vi "SFTF_attractor.vi"(10 "Target_Flash_Order":i64[](array[numeric]), 11 "Brain_EEG":dbl[][](array[numeric])) -> (2 "Non STFT":dbl[](array[numeric]), 3 "STFT Spectrogram {X}":dbl[][](array[numeric]))   [LabVIEW 2014]
uses:
  <vilib>/Analysis/3filter.llb/Filter Passband Type.ctl
  <vilib>/Analysis/4window.llb/windowTd.ctl
  <vilib>/Analysis/3filter.llb/Butterworth Filter (DBL).vi
  <vilib>/Analysis/NI_AALBase.lvlib
  <vilib>/gmath/NI_Gmath.lvlib
  <vilib>/Analysis/NI_AALPro.lvlib
panel:
  out "size(s)":i32
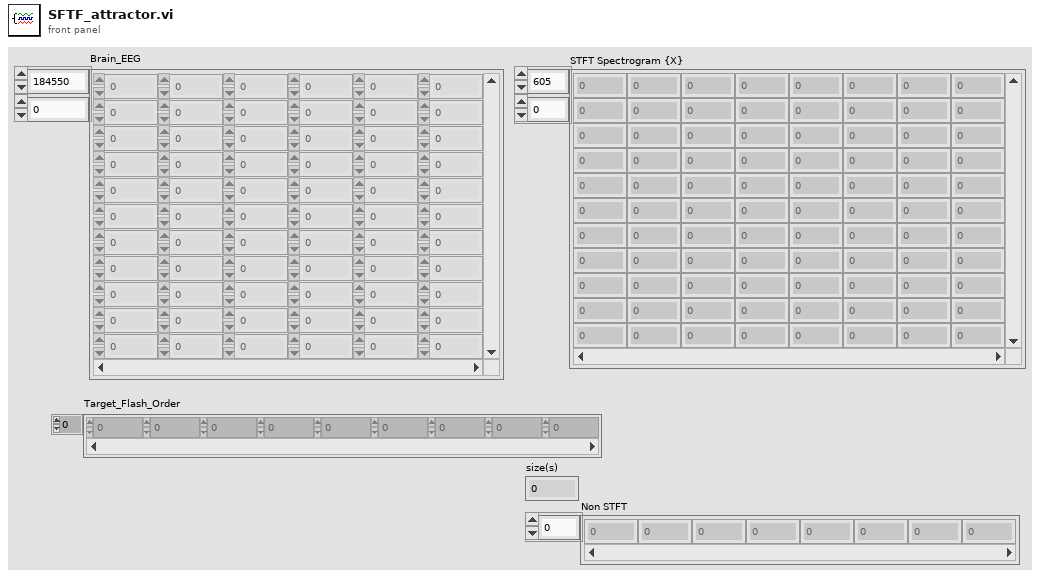
[diagram p1: front panel]
types:
  T1 = typedef "NI_AALPro.lvlib/windowTd.ctl" = u32
  T2 = typedef "NI_AALBase.lvlib/Filter Passband Type.ctl" = enum32{"Lowpass", "Highpass", "Bandpass", "Bandstop"}
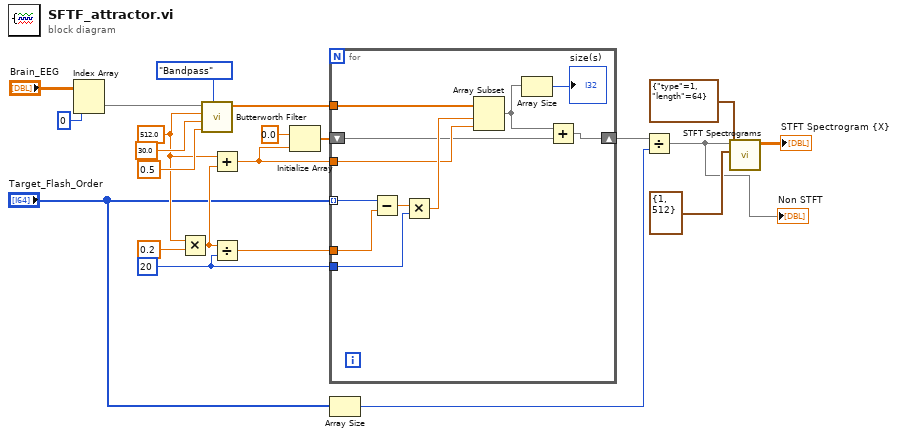
[diagram p0: block diagram]
diagram:
  w14 = 20 ("high cutoff freq: fh")
  w13 = 512.0 ("high cutoff freq: fh")
  n1 = Index Array(array="Brain_EEG", index (col)=0 ("disabled index (col)")) -> (element=w17:dbl[])  [unwired: 1 in]
  n2 = Multiply(x=w13, y=0.2) -> (x*y=w12:dbl)
  n3 = call-poly <vilib>:"Butterworth Filter.vi"("filter type"=Filter_Passband_Type."Bandpass", "low cutoff freq: fl"=0.5, "high cutoff freq: fh"=30.0, "sampling freq: fs"=w13, "X"=w17) -> ("Filtered X"=w2:dbl[])  [unwired: 3 in, 1 out]
  n4 = Add(x=w13, y=w12) -> (x+y=w10:dbl)
  n5 = Divide(x=w12, y=w14) -> (x/y=w15:dbl)
  n6 = Initialize Array(0.0 ("element"), w10) -> (w9:dbl[])
  n7 = for {
    tunnel: w2 -> [w31]
    tunnel: "Target_Flash_Order" -> [w30] mode=indexing
    tunnel: w15 -> [w29]
    tunnel: w14 -> [w28]
    tunnel: w10 -> [w27]
    shift-right: [w25] -> w8
    shift-left: w9 -> [w26]
    n8 = Subtract(x=w30, y=w29) -> (x-y=w33:dbl)
    n9 = Multiply(x=w33, y=w28) -> (x*y=w32:dbl)
    n10 = Array Subset(array=w31, index=w32, length=w27) -> (w23:dbl[])
    n11 = Array Size(array=w23) -> (size(s)=→"size(s)":i32)
    n12 = Add(x=w23, y=w26) -> (x+y=w25:dbl[])
  }
  n13 = Array Size(array="Target_Flash_Order") -> (size(s)=w7:i32)
  n14 = Divide(x=w8, y=w7) -> (x/y=w1:dbl[])
  "Non STFT" <- w1
  n15 = call <vilib>:"STFT Spectrograms.vi"("window info"=cluster{"type":T1, "length":i32} {"type"=1, "length"=64}, "time-freq sampling info"=cluster{"time steps":i32, "frequency bins":i32} {"time steps"=1, "frequency bins"=512}, "X"=w1) -> ("STFT Spectrogram {X}"=→"STFT Spectrogram {X}":dbl[][])  [unwired: 7 in, 1 out]
